vi "test Detect Changed Indices (Integer).vi"(8 "error in (no error)":errorcluster, 11 "TestCase in":refnum<class "Shared VIs.lvclass">) -> (0 "error out":errorcluster, 3 "TestCase out":refnum<class "Shared VIs.lvclass">)   [LabVIEW 2024, in "Shared VIs.lvclass"]
uses:
  Shared VIs.lvclass
  c8128e39-ba4a-4d39-8bf0-919f2f8f5ee1.vi
  f757781e-0541-4624-9f36-0c3754dd0849.vi
  <vilib>/addons/_JKI Toolkits/VI Tester/TestCase.llb/TestCase.lvclass
  C:/Program Files/National Instruments/LabVIEW 2024/vi.lib/addons/_JKI Toolkits/VI Tester/TestCase.llb/TestCase.lvclass
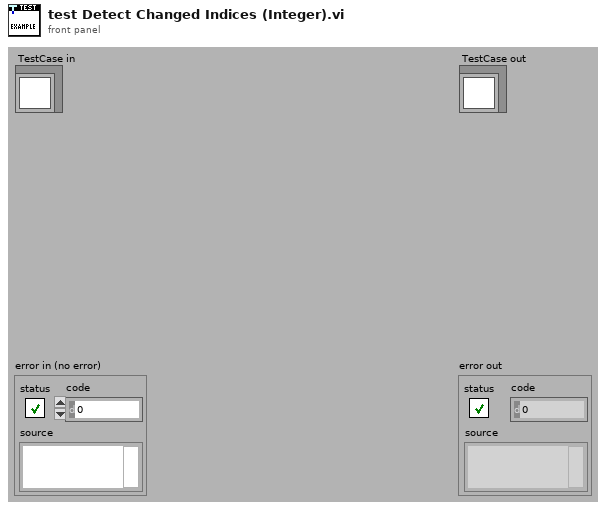
[diagram p1: front panel]
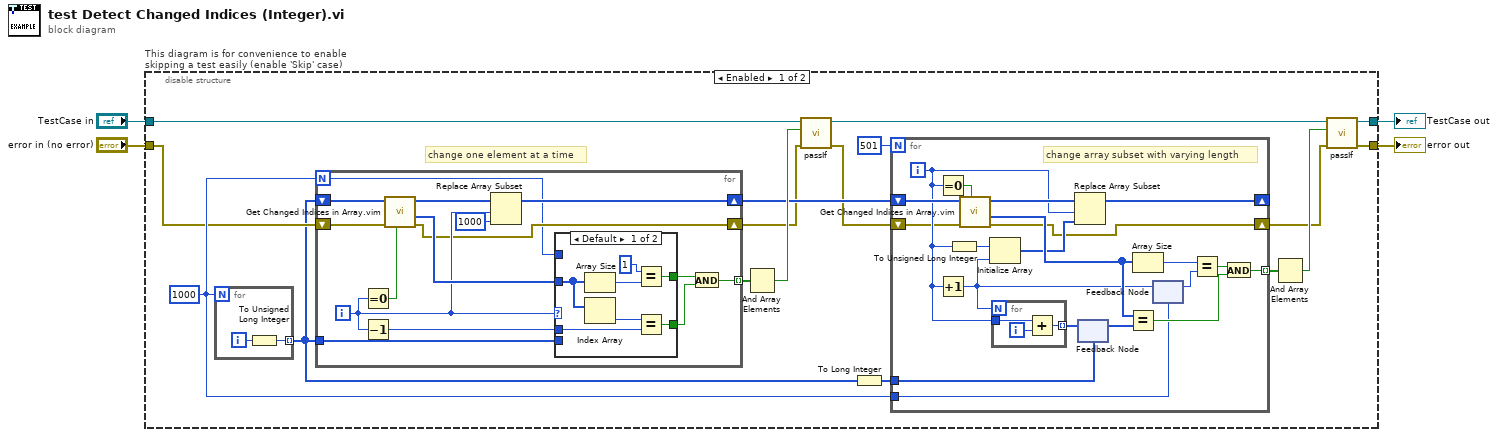
[diagram p0: block diagram]
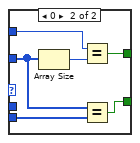
[diagram p2: hidden frame]
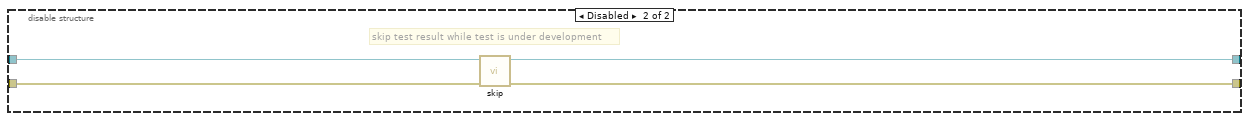
[diagram p3: hidden frame]
diagram:
  n1 = disable-structure "This diagram is for convenience to enable skipping a test easily (enable 'Skip' case)" shown="Enabled" {
    disable-tunnel: "TestCase in" -> [w21 w78]
    disable-tunnel: [w11 w76] -> w1
    disable-tunnel: [w12 w77] -> w3
    disable-tunnel: "error in (no error)" -> [w9 w75]
    frame Enabled {
      w17 = 1000
      # "change one element at a time"
      n2 = for {
        N: w17 -> [_]
        tunnel: [w73] -> w6 mode=indexing
        i -> [w74]
        n3 = To Unsigned Long Integer(number=w74) -> (unsigned 32bit integer=w73:u32)
      }
      n4 = for {
        N: w17 -> [w45]
        shift-right: [w56] -> w18
        shift-left: w6 -> [w59]
        tunnel: w6 -> [w53]
        tunnel: [w50] -> w20 mode=indexing
        shift-right: [w46] -> w10
        shift-left: w9 -> [w47]
        i -> [w48]
        n5 = Equal To 0?(x=w48) -> (x = 0?=w58:bool)
        n6 = Decrement(x=w48) -> (x-1=w49:i32)
        n7 = call "Get Changed Indices in Array.vim"("reset"=w58, "error in"=w47, "data in"=w59) -> ("error out"=w46:errorcluster, "changed indices"=w54:i32[], "data out"=w57:u32[])  [unwired: 4 in]
        n8 = Replace Array Subset(array=w57, new element=u32 1000 ("new element/subarray"), index=w48) -> (w56:u32[])
        n9 = case shown="Default" w48 {
          tunnel: w54 -> [w64 w70]
          tunnel: w45 -> [_ w71]
          tunnel: w53 -> [_ w69]
          tunnel: [w61 w68] -> w52
          tunnel: [w60 w67] -> w51
          tunnel: w49 -> [w65 _]
          frame Default {
            n10 = Array Size(array=w64) -> (size(s)=w63:i32)
            n11 = Index Array(array=w64) -> (element=w66:i32)  [unwired: 1 in]
            n12 = Equal?(x=1 ("y"), y=w63) -> (x = y?=w60:bool)
            n13 = Equal?(x=w66, y=w65) -> (x = y?=w61:bool)
          }
          frame 0 {
            n14 = Array Size(array=w70) -> (size(s)=w72:i32)
            n15 = Equal?(x=w71, y=w72) -> (x = y?=w67:bool)
            n16 = Equal?(x=w70, y=w69) -> (x = y?=w68:bool)
          }
        }
        n17 = And(x=w51, y=w52) -> (x .and. y?=w50:bool)
      }
      n18 = And Array Elements(Boolean array=w20) -> (logical AND=w19:bool)
      n19 = call-dynamic "passIf.vi"("error in (no error)"=w10, "pass"=w19, "TestCase in"=w21) -> ("error out"=w8:errorcluster, "TestCase out"=w13:refnum<class "Shared VIs.lvclass">)  [unwired: 7 in]
      n20 = To Long Integer(number=w6) -> (32bit integer=w5:i32[])
      n21 = for {
        N: 501 -> [_]
        shift-right: [w38] -> _
        shift-left: w18 -> [w41]
        tunnel: w17 -> [w27]
        tunnel: [w34] -> w14 mode=indexing
        tunnel: w5 -> [w28]
        shift-right: [w23] -> w7
        shift-left: w8 -> [w24]
        i -> [w31]
        # "change array subset with varying length"
        n22 = Equal To 0?(x=w31) -> (x = 0?=w40:bool)
        n23 = Increment(x=w31) -> (x+1=w26:i32)
        n24 = To Unsigned Long Integer(number=w31) -> (unsigned 32bit integer=w22:u32)
        n25 = call "Get Changed Indices in Array.vim"("reset"=w40, "error in"=w24, "data in"=w41) -> ("error out"=w23:errorcluster, "changed indices"=w37:i32[], "data out"=w39:u32[])  [unwired: 4 in]
        n26 = Initialize Array(w22, w26) -> (w33:u32[])
        n27 = for {
          N: w26 -> [_]
          tunnel: w31 -> [w43]
          tunnel: [w42] -> w30 mode=indexing
          i -> [w44]
          n28 = Add(x=w43, y=w44) -> (x+y=w42:i32)
        }
        n29 = Replace Array Subset(array=w39, new element=w33, index=w31) -> (w38:u32[])
        n30 = feedback #1(w28) -> (w29:i32[])
        n31 = feedback-in #1(w30) -> ()
        n32 = Equal?(x=w37, y=w29) -> (x = y?=w36:bool)
        n33 = Array Size(array=w37) -> (size(s)=w25:i32)
        n34 = feedback-in #2(w26) -> ()
        n35 = feedback #2(w27) -> (w32:i32)
        n36 = Equal?(x=w25, y=w32) -> (x = y?=w35:bool)
        n37 = And(x=w35, y=w36) -> (x .and. y?=w34:bool)
      }
      n38 = And Array Elements(Boolean array=w14) -> (logical AND=w15:bool)
      n39 = call-dynamic "passIf.vi"("error in (no error)"=w7, "pass"=w15, "TestCase in"=w13) -> ("error out"=w12:errorcluster, "TestCase out"=w11:refnum<class "Shared VIs.lvclass">)  [unwired: 7 in]
    }
    frame Disabled {
      # "skip test result while test is under development"
      n40 = call <vilib>:"skip.vi"("error in (no error)"=w75, "TestCase in"=w78) -> ("error out"=w77:errorcluster, "TestCase out"=w76:refnum<class "Shared VIs.lvclass">)  [unwired: 8 in]
    }
  }
  "error out" <- w3
  "TestCase out" <- w1
